vi "Set MultiFrame Subdiagram Label.vi"(8 "error in (no error)":errorcluster, 9 "QD Combo Box Ref":refnum<vi>, 10 "Shift Not Pressed?":bool, 11 "MultiFrame in":refnum<vi>) -> (0 "error out":errorcluster)   [LabVIEW 2017]
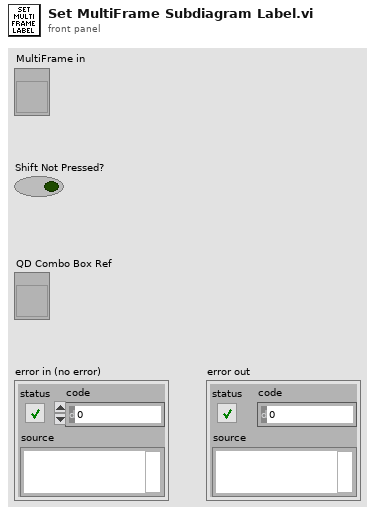
[diagram p1: front panel]
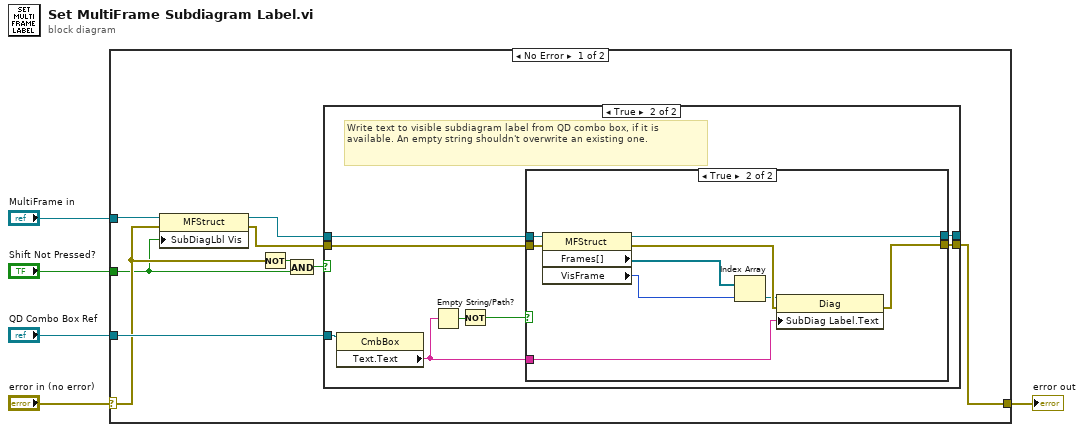
[diagram p0: block diagram]
diagram:
  n1 = case shown="No Error" "error in (no error)" {
    selector: "error in (no error)" -> [w8 w36]
    tunnel: [w11 w36] -> w5
    tunnel: "Shift Not Pressed?" -> [w6 _]
    tunnel: "QD Combo Box Ref" -> [w14 _]
    tunnel: "MultiFrame in" -> [w9 _]
    frame No Error {
      n2 = property class="MFStruct"(reference=w9, error in=w8, "SubDiagLbl Vis"=w6) -> (reference out=w10:refnum<vi>, error out=w7:errorcluster)
      n3 = Not(x=w8) -> (.not. x?=w13:bool)
      n4 = And(x=w13, y=w6) -> (x .and. y?=w12:bool)
      n5 = case shown="True" w12 {
        tunnel: w14 -> [_ w24]
        tunnel: w10 -> [w16 w18]
        tunnel: [w16 w23] -> _
        tunnel: [w15 w22] -> w11
        tunnel: w7 -> [w15 w17]
        frame False {
        }
        frame True {
          # "Write text to visible subdiagram label from QD combo box, if it is available. An empty string shouldn't overwrite an existing one."
          n6 = property class="CmbBox"(reference=w24) -> ("Text.Text"=w21:string)  [unwired: 1 in, 2 out]
          n7 = Empty String/Path?(string/path=w21) -> (empty?=w19:bool)
          n8 = Not(x=w19) -> (.not. x?=w20:bool)
          n9 = case shown="True" w20 {
            tunnel: [w26 w29] -> w23
            tunnel: [w25 w35] -> w22
            tunnel: w17 -> [w25 w34]
            tunnel: w18 -> [w26 w31]
            tunnel: w21 -> [_ w33]
            frame False {
            }
            frame True {
              n10 = property class="MFStruct"(reference=w31, error in=w34) -> (reference out=w29:refnum<vi>, error out=w32:errorcluster, "Frames[]"=w30:refnum<vi>[], "VisFrame"=w27:u32)
              n11 = Index Array(array=w30, index=w27) -> (element=w28:refnum<vi>)
              n12 = property class="Diag"(reference=w28, error in=w32, "SubDiag Label.Text"=w33) -> (error out=w35:errorcluster)  [unwired: 1 out]
            }
          }
        }
      }
    }
    frame Error {
    }
  }
  "error out" <- w5
